vi "read_plc_datasocket.vi"() -> ()   [LabVIEW 2011]
panel:
  out "LB201_B218_ST901":string
  out "LB201_B218_ST902":string
  out "LB201_B218_SV401":string
  out "LB201_B218_GN501":string
  out "LB201_B218_GQ101":string
  out "LB201_B218_GT101":string
  out "LB201_B226_GT402":string
  out "LB201_B226_GP102":string
  out "LB201_B226_GT401":string
  out "LB201_B226_GP101":string
  out "LB201_B226_GT301":string
  out "LB201_B226_U201":string
  out "LB201_B226_GT101":string
  out "KB3_B226_U201":string
  out "KB3_B226_GT401":string
  out "KB3_B226_GP101":string
  out "KB3_B226_GT101":string
  out "VS201_B226_GT301":string
  out "VS201_B226_GP101":string
  out "VS201_B226_GT401":string
  out "VS201_B226_GT101":string
  out "VS201_B226_U201":string
  out "Elapsed Time":dbl
  out "Command":string
  out "Up Time":string
  out "Startup Time":string
  out "Version":string
  out "LB201_B230_SV201":string
  out "LB201_B230_SV401":string
  out "LB201_B230_ST902":string
  out "LB201_B230_ST901":string
  out "LB201_A213_SV201":string
  out "LB201_A213_ST902":string
  out "LB201_A235_SV401":string
  out "LB201_A235_SV201":string
  out "LB201_A235_ST902":string
  out "LB201_A235_ST901":string
  out "LB201_A225_SV401":string
  out "LB201_A225_SV201":string
  out "LB201_A225_ST902":string
  out "LB201_A225_ST901":string
  out "LB201_A213_SV401":string
  out "LB201_A213_ST901":string
  out "LB201_B230_GQ101":string
  out "LB201_B230_GT101":string
  out "LB201_A235_GQ101":string
  out "LB201_A235_GT101":string
  out "LB201_B230_GN501":string
  out "LB201_A235_GN501":string
  out "LB201_A225_GT101":string
  out "LB201_A225_GQ101":string
  out "LB201_A225_GN501":string
  out "LB201_A213_GT101":string
  out "LB201_A213_GQ101":string
  out "LB201_A213_GN501":string
  out "Deque error":errorcluster
  out "DataSocket error":errorcluster
  out "# Sent Data":u64
  # "OPC Server Status"
  # "PLC Sensing Values (Per Room)"
  # "PLC Sensing Values (Common)"
  # "PLC Actuation Values"
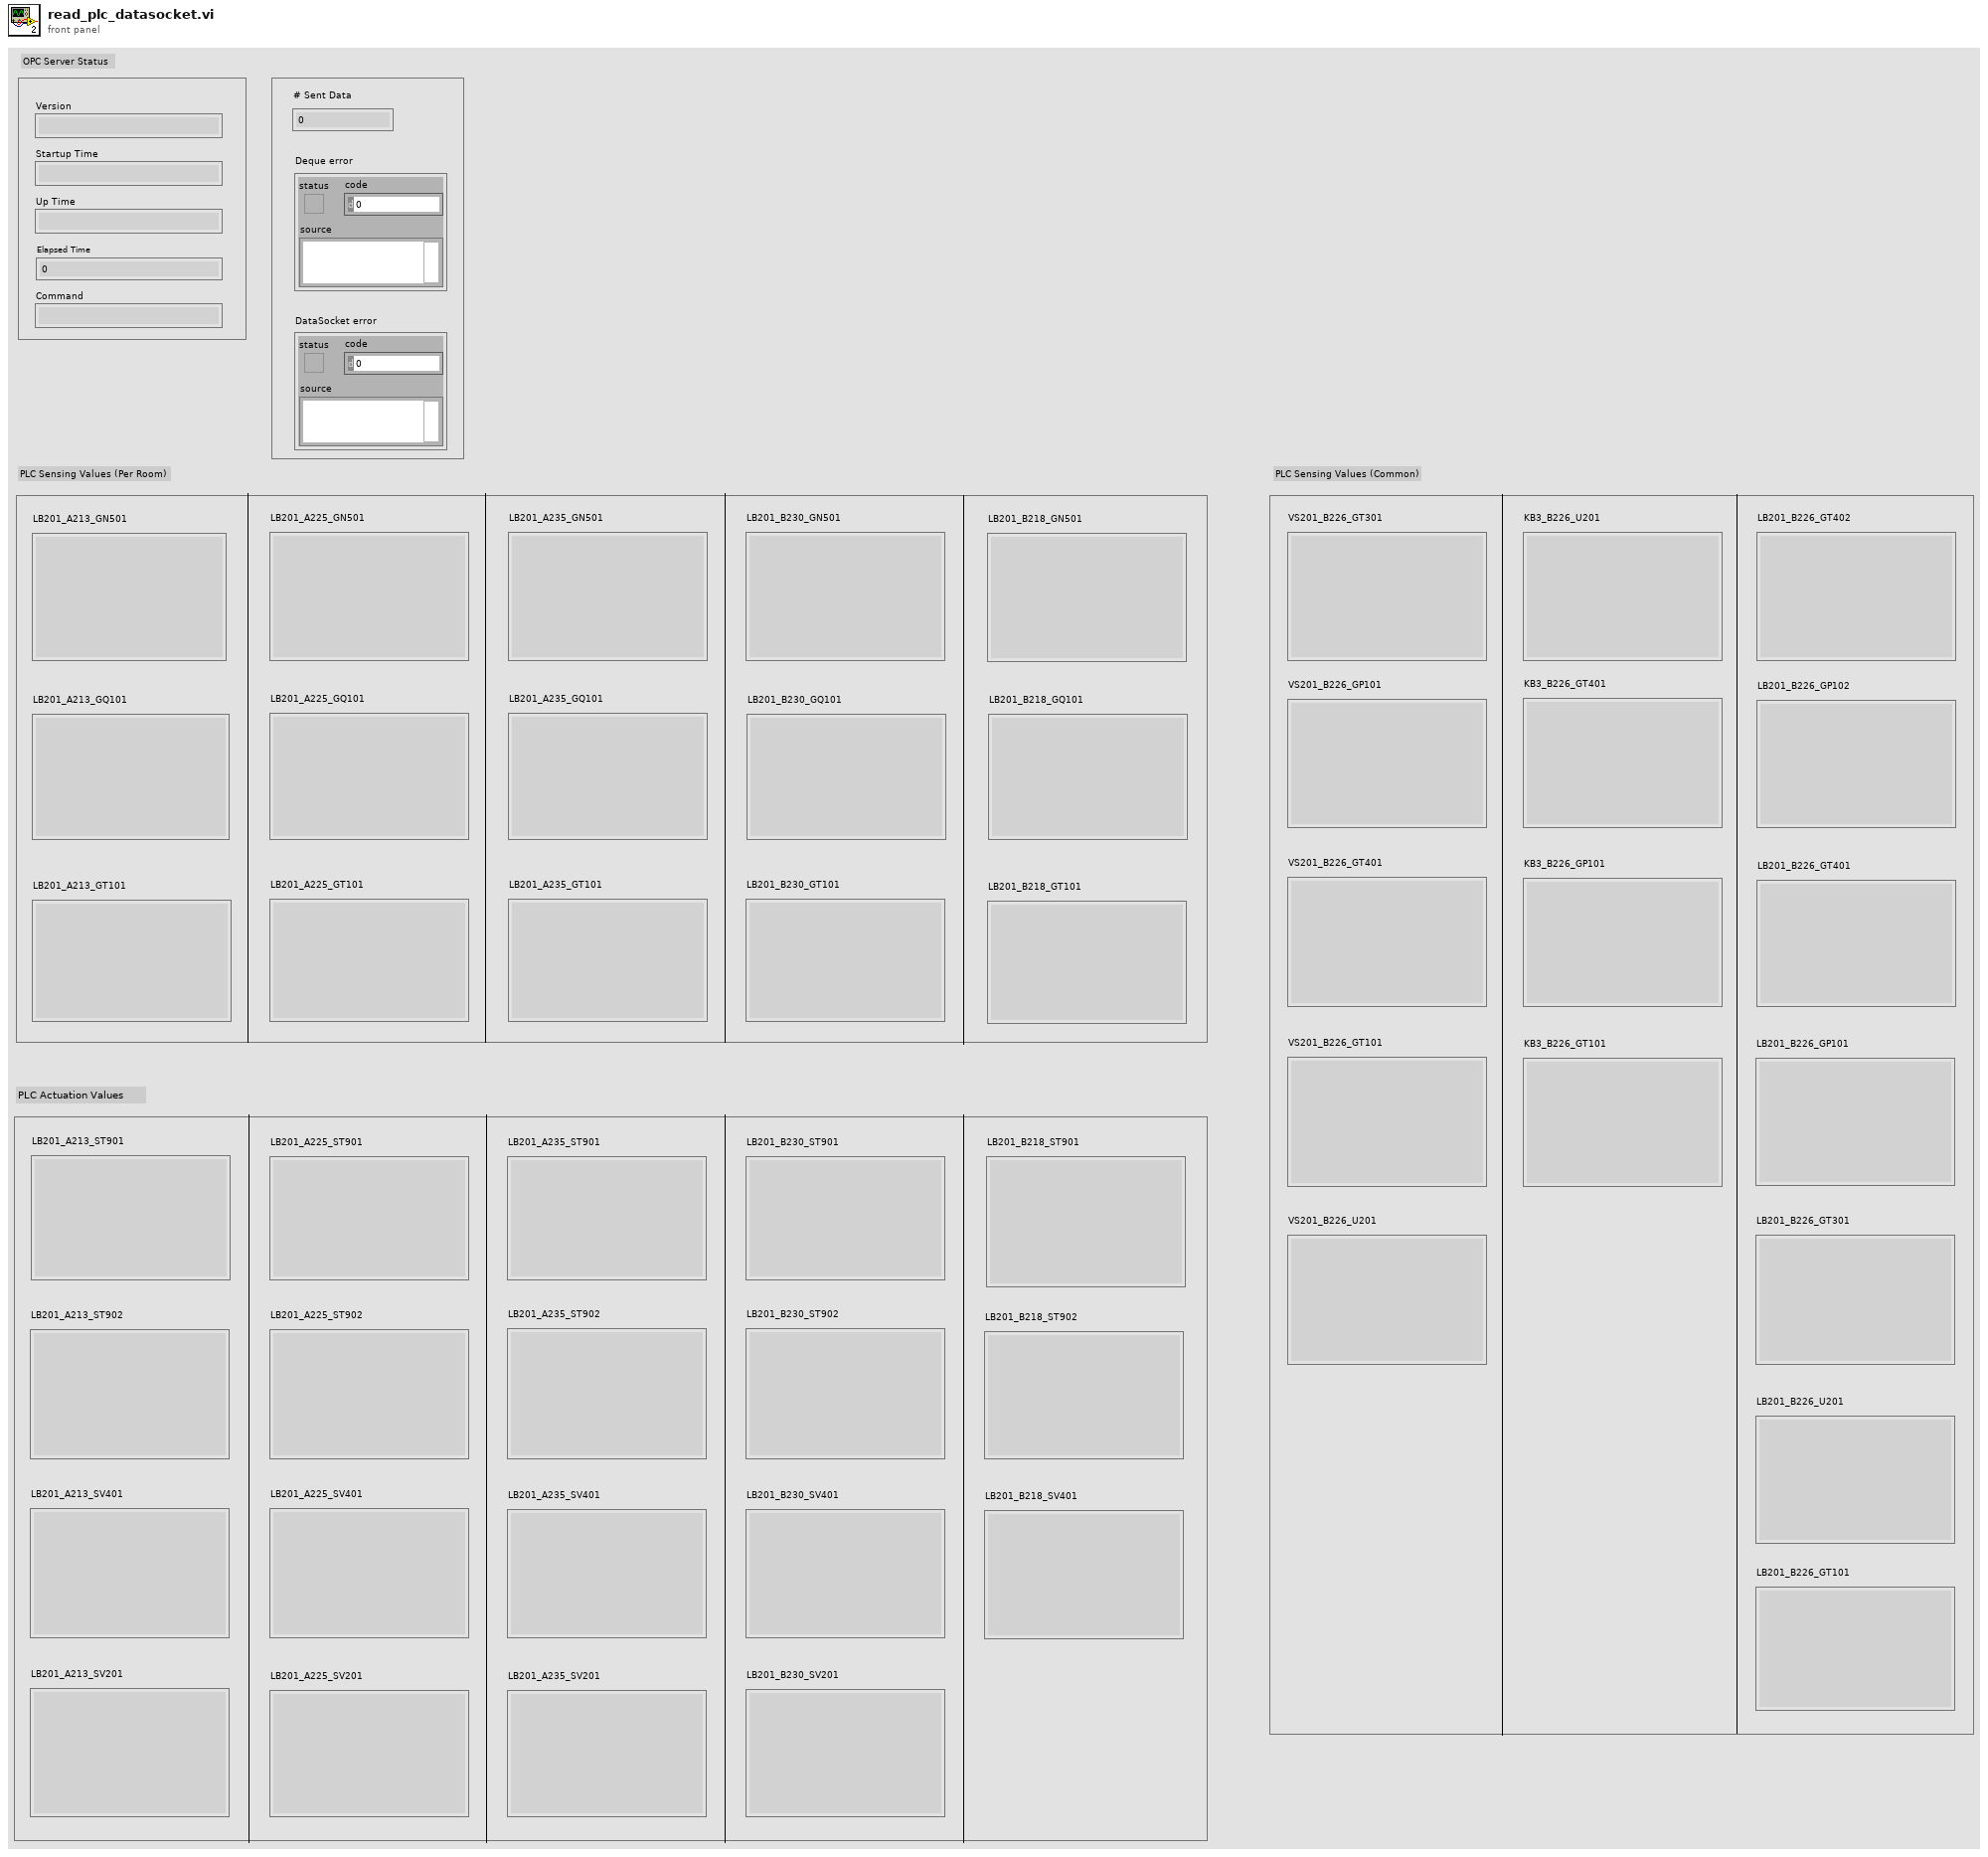
[diagram p1: front panel]
types:
  T1 = enum16{"Read", "Write", "ReadWrite", "BufferedRead", "BufferedReadWrite"}
diagram:
  w3 = string[] ["opc://localhost/Fidelix.FdxOPC/AS_KTH.AI.VS201_B226_GT301_MV.Value", "opc://localhost/Fidelix.FdxOPC/AS_KTH.AI.VS201_B226_GP101_MV.Value", "opc://localhost/Fidelix.FdxOPC/AS_KTH.AI.VS201_B226_GT401_MV.Value", "opc://localhost/Fidelix.FdxOPC/AS_KTH.AI.VS201_B226_GT101_MV.Value", "opc://localhost/Fidelix.FdxOPC/AS_KTH.AI.VS201_B226_U201_SS.Value", "opc://localhost/Fidelix.FdxOPC/AS_KTH.AI.KB3_B226_U201_SS.Value", "opc://localhost/Fidelix.FdxOPC/AS_KTH.AI.KB3_B226_GT401_MV.Value", "opc://localhost/Fidelix.FdxOPC/AS_KTH.AI.KB3_B226_GP101_MV.Value", "opc://localhost/Fidelix.FdxOPC/AS_KTH.AI.KB3_B226_GT101_MV.Value", "opc://localhost/Fidelix.FdxOPC/AS_KTH.AI.LB201_B226_GT402_MV.Value", "opc://localhost/Fidelix.FdxOPC/AS_KTH.AI.LB201_B226_GP102_MV.Value", "opc://localhost/Fidelix.FdxOPC/AS_KTH.AI.LB201_B226_GT401_MV.Value", "opc://localhost/Fidelix.FdxOPC/AS_KTH.AI.LB201_B226_GP101_MV.Value", "opc://localhost/Fidelix.FdxOPC/AS_KTH.AI.LB201_B226_GT301_MV.Value", "opc://localhost/Fidelix.FdxOPC/AS_KTH.AI.LB201_B226_U201_SS.Value", "opc://localhost/Fidelix.FdxOPC/AS_KTH.AI.LB201_B226_GT101_MV.Value"]  # Predefined items
  w32 = string[] ["opc://localhost/Fidelix.FdxOPC/AS_KTH.AI.LB201_A213_ST901_SS.Value", "opc://localhost/Fidelix.FdxOPC/AS_KTH.AI.LB201_A213_ST902_SS.Value", "opc://localhost/Fidelix.FdxOPC/AS_KTH.AI.LB201_A213_SV201_SS.Value", "opc://localhost/Fidelix.FdxOPC/AS_KTH.AI.LB201_A213_SV401_SS.Value", "opc://localhost/Fidelix.FdxOPC/AS_KTH.AI.LB201_A225_ST901_SS.Value", "opc://localhost/Fidelix.FdxOPC/AS_KTH.AI.LB201_A225_ST902_SS.Value", "opc://localhost/Fidelix.FdxOPC/AS_KTH.AI.LB201_A225_SV201_SS.Value", "opc://localhost/Fidelix.FdxOPC/AS_KTH.AI.LB201_A225_SV401_SS.Value", "opc://localhost/Fidelix.FdxOPC/AS_KTH.AI.LB201_A235_ST901_SS.Value", "opc://localhost/Fidelix.FdxOPC/AS_KTH.AI.LB201_A235_ST902_SS.Value", "opc://localhost/Fidelix.FdxOPC/AS_KTH.AI.LB201_A235_SV201_SS.Value", "opc://localhost/Fidelix.FdxOPC/AS_KTH.AI.LB201_A235_SV401_SS.Value", "opc://localhost/Fidelix.FdxOPC/AS_KTH.AI.LB201_B230_ST901_SS.Value", "opc://localhost/Fidelix.FdxOPC/AS_KTH.AI.LB201_B230_ST902_SS.Value", "opc://localhost/Fidelix.FdxOPC/AS_KTH.AI.LB201_B230_SV201_SS.Value", "opc://localhost/Fidelix.FdxOPC/AS_KTH.AI.LB201_B230_SV401_SS.Value", "opc://localhost/Fidelix.FdxOPC/AS_KTH.AI.LB201_B218_ST901_SS.Value", "opc://localhost/Fidelix.FdxOPC/AS_KTH.AI.LB201_B218_ST902_SS.Value", "opc://localhost/Fidelix.FdxOPC/AS_KTH.AI.LB201_B218_SV401_SS.Value"]  # Predefined items
  w37 = string[] ["opc://localhost/Fidelix.FdxOPC/AS_KTH.AI.LB201_A213_GN501_I.Value", "opc://localhost/Fidelix.FdxOPC/AS_KTH.AI.LB201_A213_GQ101_MV.Value", "opc://localhost/Fidelix.FdxOPC/AS_KTH.AI.LB201_A213_GT101_MV.Value", "opc://localhost/Fidelix.FdxOPC/AS_KTH.AI.LB201_A225_GN501_I.Value", "opc://localhost/Fidelix.FdxOPC/AS_KTH.AI.LB201_A225_GQ101_MV.Value", "opc://localhost/Fidelix.FdxOPC/AS_KTH.AI.LB201_A225_GT101_MV.Value", "opc://localhost/Fidelix.FdxOPC/AS_KTH.AI.LB201_A235_GN501_I.Value", "opc://localhost/Fidelix.FdxOPC/AS_KTH.AI.LB201_A235_GQ101_MV.Value", "opc://localhost/Fidelix.FdxOPC/AS_KTH.AI.LB201_A235_GT101_MV.Value", "opc://localhost/Fidelix.FdxOPC/AS_KTH.AI.LB201_B230_GN501_I.Value", "opc://localhost/Fidelix.FdxOPC/AS_KTH.AI.LB201_B230_GQ101_MV.Value", "opc://localhost/Fidelix.FdxOPC/AS_KTH.AI.LB201_B230_GT101_MV.Value", "opc://localhost/Fidelix.FdxOPC/AS_KTH.AI.LB201_B218_GN501_I.Value", "opc://localhost/Fidelix.FdxOPC/AS_KTH.AI.LB201_B218_GQ101_MV.Value", "opc://localhost/Fidelix.FdxOPC/AS_KTH.AI.LB201_B218_GT101_MV.Value"]  # Predefined items
  n1 = for {
    tunnel: w37 -> [w48] mode=indexing
    tunnel: [w47] -> w36 mode=indexing
    tunnel: [w46] -> w35 mode=indexing
    n2 = DataSocket Open(10:T1."Read" ("mode"), 11:w48) -> (0:w46:errorcluster, 3:w47:refnum<k13>)  [unwired: 1 in, 1 out]
  }
  n3 = DataSocket Open(10:T1."Read" ("mode"), 11:"opc://localhost/Fidelix.FdxOPC/ServerStatus.Version" ("URL")) -> (0:w16:errorcluster, 3:w17:refnum<k13>)  [unwired: 1 in, 1 out]
  n4 = DataSocket Open(10:T1."Read" ("mode"), 11:"opc://localhost/Fidelix.FdxOPC/ServerStatus.StartupTime" ("URL")) -> (0:w14:errorcluster, 3:w15:refnum<k13>)  [unwired: 1 in, 1 out]
  n5 = DataSocket Open(10:T1."Read" ("mode"), 11:"opc://localhost/Fidelix.FdxOPC/ServerStatus.UpTime" ("URL")) -> (0:w12:errorcluster, 3:w13:refnum<k13>)  [unwired: 1 in, 1 out]
  n6 = DataSocket Open(10:T1."Read" ("mode"), 11:"opc://localhost/Fidelix.FdxOPC/ServerStatus.ElapsedTime" ("URL")) -> (0:w10:errorcluster, 3:w11:refnum<k13>)  [unwired: 1 in, 1 out]
  n7 = DataSocket Open(10:T1."Read" ("mode"), 11:"opc://localhost/Fidelix.FdxOPC/ServerStatus.Command" ("URL")) -> (0:w8:errorcluster, 3:w9:refnum<k13>)  [unwired: 1 in, 1 out]
  n8 = while {
    tunnel: w17 -> [w58]
    tunnel: w16 -> [w57]
    tunnel: w15 -> [w56]
    tunnel: w14 -> [w55]
    tunnel: w13 -> [w54]
    tunnel: w12 -> [w53]
    tunnel: w11 -> [w52]
    tunnel: w10 -> [w51]
    tunnel: w9 -> [w50]
    tunnel: w8 -> [w49]
    stop <- TRUE continue-if-true
    n9 = DataSocket Read(8:w57, 9:100 ("ms timeout (10000)"), 10:"", 11:w58) -> (2:→"Version":string)  [unwired: 7 out]
    n10 = DataSocket Read(8:w55, 9:100 ("ms timeout (10000)"), 10:"", 11:w56) -> (2:→"Startup Time":string)  [unwired: 7 out]
    n11 = DataSocket Read(8:w53, 9:100 ("ms timeout (10000)"), 10:"", 11:w54) -> (2:→"Up Time":string)  [unwired: 7 out]
    n12 = DataSocket Read(8:w51, 9:100 ("ms timeout (10000)"), 10:0.0, 11:w52) -> (2:→"Elapsed Time":dbl)  [unwired: 7 out]
    n13 = DataSocket Read(8:w49, 9:100 ("ms timeout (10000)"), 10:"", 11:w50) -> (2:→"Command":string)  [unwired: 7 out]
    n14 = Wait Until Next ms Multiple(millisecond multiple=u32 1000) -> ()  [unwired: 1 out]
  }
  n15 = Obtain Queue(max queue size (-1, unlimited)=-1, name (unnamed)="SendingQuePLC", element data type="") -> (queue out=w2:refnum<queue>, error out=w1:errorcluster)  [unwired: 2 in, 1 out]
  n16 = while {
    tunnel: w1 -> [w322]
    tunnel: w2 -> [w321]
    tunnel: w36 -> [w250]
    tunnel: w35 -> [w249]
    tunnel: [w247] -> w34
    tunnel: [w246] -> w33
    stop <- TRUE continue-if-true
    w117 = "\r"
    w116 = "\r"
    w115 = "\r"
    w142 = "\r"
    w154 = "\r"
    w166 = "\r"
    w178 = "\r"
    w190 = "\r"
    w125 = "\r"
    w126 = "\r"
    w127 = "\r"
    w128 = "\r"
    w129 = "\r"
    w130 = "\r"
    w191 = "\r"
    # "PLC Sensing Values (Per Room)"
    n17 = for {
      tunnel: w250 -> [w328] mode=indexing
      tunnel: [w330] -> w247 mode=indexing
      tunnel: w249 -> [w327] mode=indexing
      tunnel: [w325] -> w248 mode=indexing
      tunnel: [w329] -> w246 mode=indexing
      n18 = DataSocket Read(8:w327, 9:500 ("ms timeout (10000)"), 10:0.0, 11:w328) -> (0:w329:errorcluster, 2:w325:dbl, 3:w330:refnum<k13>)  [unwired: 5 out]
    }
    n19 = Build Array(w248) -> (w118:dbl[][])
    n20 = Index Array(array=w118, index (row)=0, index (col)=12 ("disabled index (col)")) -> (element=w78:dbl)
    n21 = Index Array(array=w118, index (row)=0, index (col)=13 ("disabled index (col)")) -> (element=w77:dbl)
    n22 = Index Array(array=w118, index (row)=0, index (col)=14 ("disabled index (col)")) -> (element=w76:dbl)
    n23 = Index Array(array=w118, index (row)=0, index (col)=0 ("disabled index (col)")) -> (element=w237:dbl)
    n24 = Index Array(array=w118, index (row)=0, index (col)=1 ("disabled index (col)")) -> (element=w179:dbl)
    n25 = Index Array(array=w118, index (row)=0, index (col)=2 ("disabled index (col)")) -> (element=w167:dbl)
    n26 = Index Array(array=w118, index (row)=0, index (col)=3 ("disabled index (col)")) -> (element=w155:dbl)
    n27 = Index Array(array=w118, index (row)=0, index (col)=4 ("disabled index (col)")) -> (element=w143:dbl)
    n28 = Index Array(array=w118, index (row)=0, index (col)=5 ("disabled index (col)")) -> (element=w131:dbl)
    n29 = Index Array(array=w118, index (row)=0, index (col)=6 ("disabled index (col)")) -> (element=w220:dbl)
    n30 = Index Array(array=w118, index (row)=0, index (col)=7 ("disabled index (col)")) -> (element=w219:dbl)
    n31 = Index Array(array=w118, index (row)=0, index (col)=8 ("disabled index (col)")) -> (element=w218:dbl)
    n32 = Index Array(array=w118, index (row)=0, index (col)=9 ("disabled index (col)")) -> (element=w217:dbl)
    n33 = Index Array(array=w118, index (row)=0, index (col)=10 ("disabled index (col)")) -> (element=w216:dbl)
    n34 = Index Array(array=w118, index (row)=0, index (col)=11 ("disabled index (col)")) -> (element=w215:dbl)
    n35 = Wait Until Next ms Multiple(millisecond multiple=u32 30000) -> ()  [unwired: 1 out]
    n36 = Number To Fractional String(number=w143, precision (6)=i16 2) -> (F-format string=w146:string)  [unwired: 2 in]
    n37 = Number To Fractional String(number=w167, precision (6)=i16 2) -> (F-format string=w170:string)  [unwired: 2 in]
    n38 = Format Date/Time String(time format string (%c)="%y%m%d%H%M%S") -> (date/time string=w171:string)  [unwired: 2 in]
    n39 = Number To Fractional String(number=w179, precision (6)=i16 2) -> (F-format string=w182:string)  [unwired: 2 in]
    n40 = Format Date/Time String(time format string (%c)="%y%m%d%H%M%S") -> (date/time string=w183:string)  [unwired: 2 in]
    n41 = Number To Fractional String(number=w131, precision (6)=i16 2) -> (F-format string=w134:string)  [unwired: 2 in]
    n42 = Number To Fractional String(number=w155, precision (6)=i16 2) -> (F-format string=w158:string)  [unwired: 2 in]
    n43 = Format Date/Time String(time format string (%c)="%y%m%d%H%M%S") -> (date/time string=w159:string)  [unwired: 2 in]
    n44 = Number To Fractional String(number=w237, precision (6)=i16 2) -> (F-format string=w317:string)  [unwired: 2 in]
    n45 = Format Date/Time String(time format string (%c)="%y%m%d%H%M%S") -> (date/time string=w316:string)  [unwired: 2 in]
    n46 = Number To Fractional String(number=w220, precision (6)=i16 2) -> (F-format string=w308:string)  [unwired: 2 in]
    n47 = Number To Fractional String(number=w218, precision (6)=i16 2) -> (F-format string=w294:string)  [unwired: 2 in]
    n48 = Number To Fractional String(number=w219, precision (6)=i16 2) -> (F-format string=w285:string)  [unwired: 2 in]
    n49 = Number To Fractional String(number=w217, precision (6)=i16 2) -> (F-format string=w299:string)  [unwired: 2 in]
    n50 = Number To Fractional String(number=w78, precision (6)=i16 2) -> (F-format string=w85:string)  [unwired: 2 in]
    n51 = Number To Fractional String(number=w215, precision (6)=i16 2) -> (F-format string=w271:string)  [unwired: 2 in]
    n52 = Number To Fractional String(number=w216, precision (6)=i16 2) -> (F-format string=w280:string)  [unwired: 2 in]
    n53 = Number To Fractional String(number=w76, precision (6)=i16 2) -> (F-format string=w99:string)  [unwired: 2 in]
    n54 = Number To Fractional String(number=w77, precision (6)=i16 2) -> (F-format string=w90:string)  [unwired: 2 in]
    n55 = Format Date/Time String(time format string (%c)="%y%m%d%H%M%S") -> (date/time string=w147:string)  [unwired: 2 in]
    n56 = Format Date/Time String(time format string (%c)="%y%m%d%H%M%S") -> (date/time string=w295:string)  [unwired: 2 in]
    n57 = Format Date/Time String(time format string (%c)="%y%m%d%H%M%S") -> (date/time string=w284:string)  [unwired: 2 in]
    n58 = Format Date/Time String(time format string (%c)="%y%m%d%H%M%S") -> (date/time string=w135:string)  [unwired: 2 in]
    n59 = Format Date/Time String(time format string (%c)="%y%m%d%H%M%S") -> (date/time string=w298:string)  [unwired: 2 in]
    n60 = Format Date/Time String(time format string (%c)="%y%m%d%H%M%S") -> (date/time string=w86:string)  [unwired: 2 in]
    n61 = Format Date/Time String(time format string (%c)="%y%m%d%H%M%S") -> (date/time string=w270:string)  [unwired: 2 in]
    n62 = Format Date/Time String(time format string (%c)="%y%m%d%H%M%S") -> (date/time string=w281:string)  [unwired: 2 in]
    n63 = Format Date/Time String(time format string (%c)="%y%m%d%H%M%S") -> (date/time string=w100:string)  [unwired: 2 in]
    n64 = Format Date/Time String(time format string (%c)="%y%m%d%H%M%S") -> (date/time string=w89:string)  [unwired: 2 in]
    n65 = Format Date/Time String(time format string (%c)="%y%m%d%H%M%S") -> (date/time string=w309:string)  [unwired: 2 in]
    n66 = Concatenate Strings("2002" ("string"), w154, "C" ("string"), w154, "30" ("string"), w154, w146, w154, w147, w154, "LB201_A225", w154, "0.3145 0.3240 0.5" ("string")) -> (w144:string)
    "LB201_A225_GQ101" <- w144
    n67 = Concatenate Strings("2001" ("string"), w178, "T" ("string"), w178, "10" ("string"), w178, w170, w178, w171, w178, "LB201_A213", w178, "0.5524 0.3240 0.5" ("string")) -> (w168:string)
    "LB201_A213_GT101" <- w168
    n68 = Concatenate Strings("2001" ("string"), w190, "C" ("string"), w190, "30" ("string"), w190, w182, w190, w183, w190, "LB201_A213", w190, "0.5524 0.3240 0.5" ("string")) -> (w180:string)
    "LB201_A213_GQ101" <- w180
    n69 = Concatenate Strings("2002" ("string"), w142, "T" ("string"), w142, "10" ("string"), w142, w134, w142, w135, w142, "LB201_A225", w142, "0.3145 0.3240 0.5" ("string")) -> (w132:string)
    "LB201_A225_GT101" <- w132
    n70 = Concatenate Strings("2002" ("string"), w166, "M" ("string"), w166, "51" ("string"), w166, w158, w166, w159, w166, "LB201_A225", w166, "0.3145 0.3240 0.5" ("string")) -> (w156:string)
    "LB201_A225_GN501" <- w156
    n71 = Concatenate Strings("2001" ("string"), w191, "M" ("string"), w191, "51" ("string"), w191, w317, w191, w316, w191, "LB201_A213", w191, "0.5524 0.3240 0.5" ("string")) -> (w320:string)
    "LB201_A213_GN501" <- w320
    n72 = Concatenate Strings("2003" ("string"), w130, "M" ("string"), w130, "51" ("string"), w130, w308, w130, w309, w130, "LB201_A235", w130, "0.1735 0.3240 0.5" ("string")) -> (w305:string)
    "LB201_A235_GN501" <- w305
    n73 = Concatenate Strings("2003" ("string"), w128, "T" ("string"), w128, "10" ("string"), w128, w294, w128, w295, w128, "LB201_A235", w128, "0.1735 0.3240 0.5" ("string")) -> (w291:string)
    "LB201_A235_GT101" <- w291
    n74 = Concatenate Strings("2003" ("string"), w129, "C" ("string"), w129, "30" ("string"), w129, w285, w129, w284, w129, "LB201_A235", w129, "0.1735 0.3240 0.5" ("string")) -> (w288:string)
    "LB201_A235_GQ101" <- w288
    n75 = Concatenate Strings("2004" ("string"), w127, "M" ("string"), w127, "51" ("string"), w127, w299, w127, w298, w127, "LB201_B230", w127, "0.2761 0.6773 0.5" ("string")) -> (w302:string)
    "LB201_B230_GN501" <- w302
    n76 = Concatenate Strings("2005" ("string"), w115, "M" ("string"), w115, "51" ("string"), w115, w85, w115, w86, w115, "LB201_B218", w115, "0.5844 0.6607 0.5" ("string")) -> (w82:string)
    "LB201_B218_GN501" <- w82
    n77 = Concatenate Strings("2004" ("string"), w125, "T" ("string"), w125, "10" ("string"), w125, w271, w125, w270, w125, "LB201_B230", w125, "0.2761 0.6773 0.5" ("string")) -> (w274:string)
    "LB201_B230_GT101" <- w274
    n78 = Concatenate Strings("2004" ("string"), w126, "C" ("string"), w126, "30" ("string"), w126, w280, w126, w281, w126, "LB201_B230", w126, "0.2761 0.6773 0.5" ("string")) -> (w277:string)
    "LB201_B230_GQ101" <- w277
    n79 = Concatenate Strings("2005" ("string"), w117, "T" ("string"), w117, "10" ("string"), w117, w99, w117, w100, w117, "LB201_B218", w117, "0.5844 0.6607 0.5" ("string")) -> (w96:string)
    "LB201_B218_GT101" <- w96
    n80 = Concatenate Strings("2005" ("string"), w116, "C" ("string"), w116, "30" ("string"), w116, w90, w116, w89, w116, "LB201_B218", w116, "0.5844 0.6607 0.5" ("string")) -> (w93:string)
    "LB201_B218_GQ101" <- w93
    n81 = Enqueue Element(queue=w321, element=w320, error in (no error)=w322) -> (queue out=w314:refnum<queue>, error out=w312:errorcluster)  [unwired: 1 in, 1 out]
    n82 = Enqueue Element(queue=w314, element=w180, error in (no error)=w312) -> (queue out=w313:refnum<queue>, error out=w311:errorcluster)  [unwired: 1 in, 1 out]
    n83 = Enqueue Element(queue=w313, element=w168, error in (no error)=w311) -> (queue out=w268:refnum<queue>, error out=w267:errorcluster)  [unwired: 1 in, 1 out]
    n84 = Enqueue Element(queue=w268, element=w156, error in (no error)=w267) -> (queue out=w266:refnum<queue>, error out=w265:errorcluster)  [unwired: 1 in, 1 out]
    n85 = Enqueue Element(queue=w266, element=w144, error in (no error)=w265) -> (queue out=w264:refnum<queue>, error out=w263:errorcluster)  [unwired: 1 in, 1 out]
    n86 = Enqueue Element(queue=w264, element=w132, error in (no error)=w263) -> (queue out=w262:refnum<queue>, error out=w261:errorcluster)  [unwired: 1 in, 1 out]
    n87 = Enqueue Element(queue=w262, element=w305, error in (no error)=w261) -> (queue out=w260:refnum<queue>, error out=w259:errorcluster)  [unwired: 1 in, 1 out]
    n88 = Enqueue Element(queue=w260, element=w288, error in (no error)=w259) -> (queue out=w258:refnum<queue>, error out=w257:errorcluster)  [unwired: 1 in, 1 out]
    n89 = Enqueue Element(queue=w258, element=w291, error in (no error)=w257) -> (queue out=w256:refnum<queue>, error out=w255:errorcluster)  [unwired: 1 in, 1 out]
    n90 = Enqueue Element(queue=w256, element=w302, error in (no error)=w255) -> (queue out=w254:refnum<queue>, error out=w253:errorcluster)  [unwired: 1 in, 1 out]
    n91 = Enqueue Element(queue=w254, element=w277, error in (no error)=w253) -> (queue out=w252:refnum<queue>, error out=w251:errorcluster)  [unwired: 1 in, 1 out]
    n92 = Enqueue Element(queue=w252, element=w274, error in (no error)=w251) -> (queue out=w80:refnum<queue>, error out=w79:errorcluster)  [unwired: 1 in, 1 out]
    n93 = Enqueue Element(queue=w80, element=w82, error in (no error)=w79) -> (queue out=w102:refnum<queue>, error out=w103:errorcluster)  [unwired: 1 in, 1 out]
    n94 = Enqueue Element(queue=w102, element=w93, error in (no error)=w103) -> (queue out=w104:refnum<queue>, error out=w105:errorcluster)  [unwired: 1 in, 1 out]
    n95 = Enqueue Element(queue=w104, element=w96, error in (no error)=w105) -> ()  [unwired: 1 in, 3 out]
  }
  n96 = for {
    tunnel: w34 -> [w332] mode=indexing
    tunnel: w33 -> [w331] mode=indexing
    n97 = DataSocket Close(8:w331, 11:w332) -> ()  [unwired: 3 out]
  }
  n98 = DataSocket Open(10:T1."Write" ("mode"), 11:"dstp://localhost/plcs" ("URL 3")) -> (0:w39:errorcluster, 3:w40:refnum<k13>)  [unwired: 2 in]
  n99 = while {
    tunnel: w2 -> [w345]
    tunnel: w40 -> [w344]
    tunnel: w39 -> [w339]
    i -> [w337]
    stop <- w338 stop-if-true
    n100 = Dequeue Element(queue=w345) -> (element=w342:string, error out=w341:errorcluster)  [unwired: 2 in, 2 out]
    "Deque error" <- w341
    n101 = To Variant(anything=w342) -> (Variant=w343:variant)
    n102 = DataSocket Write(8:w339, 10:w343, 11:w344) -> (0:w340:errorcluster)  [unwired: 3 out]
    "DataSocket error" <- w340
    n103 = Unbundle By Name(w340) -> ("status"=w334:bool)
    n104 = Unbundle By Name(w341) -> ("status"=w333:bool)
    n105 = Compound Arithmetic op=OR(w334, w333) -> (w338:bool)
    n106 = call "logging.vi"("data"="counter.vi: datasocket error.", "Boolean"=w334) -> ()  [unwired: 1 in]
    n107 = call "logging.vi"("data"="counter.vi: deque error.", "Boolean"=w333) -> ()  [unwired: 1 in]
    "# Sent Data" <- w337
  }
  n108 = for {
    tunnel: w3 -> [w349] mode=indexing
    tunnel: [w348] -> w4 mode=indexing
    tunnel: [w347] -> w5 mode=indexing
    n109 = DataSocket Open(10:T1."Read" ("mode"), 11:w349) -> (0:w347:errorcluster, 3:w348:refnum<k13>)  [unwired: 1 in, 1 out]
  }
  n110 = while {
    tunnel: w4 -> [w611]
    tunnel: w5 -> [w610]
    tunnel: [w608] -> w6
    tunnel: [w607] -> w7
    tunnel: w2 -> [w565]
    tunnel: w1 -> [w564]
    stop <- TRUE continue-if-true
    w361 = "\r"
    w374 = "\r"
    w385 = "\r"
    w397 = "\r"
    w409 = "\r"
    w421 = "\r"
    w433 = "\r"
    w445 = "\r"
    w457 = "\r"
    w469 = "\r"
    w481 = "\r"
    w493 = "\r"
    w505 = "\r"
    w518 = "\r"
    w529 = "\r"
    w541 = "\r"
    # "PLC Sensing Values (Common)"
    n111 = for {
      tunnel: w611 -> [w618] mode=indexing
      tunnel: [w620] -> w608 mode=indexing
      tunnel: w610 -> [w617] mode=indexing
      tunnel: [w615] -> w609 mode=indexing
      tunnel: [w619] -> w607 mode=indexing
      n112 = DataSocket Read(8:w617, 9:500 ("ms timeout (10000)"), 10:0.0, 11:w618) -> (0:w619:errorcluster, 2:w615:dbl, 3:w620:refnum<k13>)  [unwired: 5 out]
    }
    n113 = Build Array(w609) -> (w574:dbl[][])
    n114 = Index Array(array=w574, index (row)=0, index (col)=0 ("disabled index (col)")) -> (element=w530:dbl)
    n115 = Index Array(array=w574, index (row)=0, index (col)=1 ("disabled index (col)")) -> (element=w507:dbl)
    n116 = Index Array(array=w574, index (row)=0, index (col)=2 ("disabled index (col)")) -> (element=w506:dbl)
    n117 = Index Array(array=w574, index (row)=0, index (col)=3 ("disabled index (col)")) -> (element=w494:dbl)
    n118 = Index Array(array=w574, index (row)=0, index (col)=4 ("disabled index (col)")) -> (element=w482:dbl)
    n119 = Index Array(array=w574, index (row)=0, index (col)=5 ("disabled index (col)")) -> (element=w470:dbl)
    n120 = Index Array(array=w574, index (row)=0, index (col)=6 ("disabled index (col)")) -> (element=w458:dbl)
    n121 = Index Array(array=w574, index (row)=0, index (col)=7 ("disabled index (col)")) -> (element=w446:dbl)
    n122 = Index Array(array=w574, index (row)=0, index (col)=8 ("disabled index (col)")) -> (element=w434:dbl)
    n123 = Index Array(array=w574, index (row)=0, index (col)=9 ("disabled index (col)")) -> (element=w422:dbl)
    n124 = Index Array(array=w574, index (row)=0, index (col)=10 ("disabled index (col)")) -> (element=w410:dbl)
    n125 = Index Array(array=w574, index (row)=0, index (col)=11 ("disabled index (col)")) -> (element=w398:dbl)
    n126 = Index Array(array=w574, index (row)=0, index (col)=12 ("disabled index (col)")) -> (element=w386:dbl)
    n127 = Index Array(array=w574, index (row)=0, index (col)=13 ("disabled index (col)")) -> (element=w362:dbl)
    n128 = Index Array(array=w574, index (row)=0, index (col)=14 ("disabled index (col)")) -> (element=w363:dbl)
    n129 = Index Array(array=w574, index (row)=0, index (col)=15 ("disabled index (col)")) -> (element=w350:dbl)
    n130 = Wait Until Next ms Multiple(millisecond multiple=u32 30000) -> ()  [unwired: 1 out]
    n131 = Number To Fractional String(number=w507, precision (6)=i16 2) -> (F-format string=w522:string)  [unwired: 2 in]
    n132 = Number To Fractional String(number=w530, precision (6)=i16 2) -> (F-format string=w534:string)  [unwired: 2 in]
    n133 = Number To Fractional String(number=w494, precision (6)=i16 2) -> (F-format string=w498:string)  [unwired: 2 in]
    n134 = Number To Fractional String(number=w506, precision (6)=i16 2) -> (F-format string=w511:string)  [unwired: 2 in]
    n135 = Number To Fractional String(number=w482, precision (6)=i16 2) -> (F-format string=w486:string)  [unwired: 2 in]
    n136 = Number To Fractional String(number=w458, precision (6)=i16 2) -> (F-format string=w462:string)  [unwired: 2 in]
    n137 = Number To Fractional String(number=w470, precision (6)=i16 2) -> (F-format string=w474:string)  [unwired: 2 in]
    n138 = Number To Fractional String(number=w434, precision (6)=i16 2) -> (F-format string=w438:string)  [unwired: 2 in]
    n139 = Number To Fractional String(number=w446, precision (6)=i16 2) -> (F-format string=w450:string)  [unwired: 2 in]
    n140 = Number To Fractional String(number=w410, precision (6)=i16 2) -> (F-format string=w414:string)  [unwired: 2 in]
    n141 = Number To Fractional String(number=w422, precision (6)=i16 2) -> (F-format string=w426:string)  [unwired: 2 in]
    n142 = Number To Fractional String(number=w398, precision (6)=i16 2) -> (F-format string=w402:string)  [unwired: 2 in]
    n143 = Number To Fractional String(number=w386, precision (6)=i16 2) -> (F-format string=w390:string)  [unwired: 2 in]
    n144 = Number To Fractional String(number=w350, precision (6)=i16 2) -> (F-format string=w355:string)  [unwired: 2 in]
    n145 = Number To Fractional String(number=w362, precision (6)=i16 2) -> (F-format string=w379:string)  [unwired: 2 in]
    n146 = Number To Fractional String(number=w363, precision (6)=i16 2) -> (F-format string=w368:string)  [unwired: 2 in]
    n147 = Format Date/Time String(time format string (%c)="%y%m%d%H%M%S") -> (date/time string=w521:string)  [unwired: 2 in]
    n148 = Format Date/Time String(time format string (%c)="%y%m%d%H%M%S") -> (date/time string=w533:string)  [unwired: 2 in]
    n149 = Format Date/Time String(time format string (%c)="%y%m%d%H%M%S") -> (date/time string=w497:string)  [unwired: 2 in]
    n150 = Format Date/Time String(time format string (%c)="%y%m%d%H%M%S") -> (date/time string=w510:string)  [unwired: 2 in]
    n151 = Format Date/Time String(time format string (%c)="%y%m%d%H%M%S") -> (date/time string=w485:string)  [unwired: 2 in]
    n152 = Format Date/Time String(time format string (%c)="%y%m%d%H%M%S") -> (date/time string=w461:string)  [unwired: 2 in]
    n153 = Format Date/Time String(time format string (%c)="%y%m%d%H%M%S") -> (date/time string=w473:string)  [unwired: 2 in]
    n154 = Format Date/Time String(time format string (%c)="%y%m%d%H%M%S") -> (date/time string=w437:string)  [unwired: 2 in]
    n155 = Format Date/Time String(time format string (%c)="%y%m%d%H%M%S") -> (date/time string=w449:string)  [unwired: 2 in]
    n156 = Format Date/Time String(time format string (%c)="%y%m%d%H%M%S") -> (date/time string=w413:string)  [unwired: 2 in]
    n157 = Format Date/Time String(time format string (%c)="%y%m%d%H%M%S") -> (date/time string=w425:string)  [unwired: 2 in]
    n158 = Format Date/Time String(time format string (%c)="%y%m%d%H%M%S") -> (date/time string=w401:string)  [unwired: 2 in]
    n159 = Format Date/Time String(time format string (%c)="%y%m%d%H%M%S") -> (date/time string=w389:string)  [unwired: 2 in]
    n160 = Format Date/Time String(time format string (%c)="%y%m%d%H%M%S") -> (date/time string=w354:string)  [unwired: 2 in]
    n161 = Format Date/Time String(time format string (%c)="%y%m%d%H%M%S") -> (date/time string=w378:string)  [unwired: 2 in]
    n162 = Format Date/Time String(time format string (%c)="%y%m%d%H%M%S") -> (date/time string=w367:string)  [unwired: 2 in]
    n163 = Concatenate Strings("2000" ("string"), w529, "P" ("string"), w529, "507" ("string"), w529, w522, w529, w521, w529, "VS201_B226", w529, "0.4619 0.6696 0.5" ("string")) -> (w519:string)
    "VS201_B226_GP101" <- w519
    n164 = Concatenate Strings("2000" ("string"), w541, "T" ("string"), w541, "19" ("string"), w541, w534, w541, w533, w541, "VS201_B226", w541, "0.4619 0.6696 0.5" ("string")) -> (w531:string)
    "VS201_B226_GT301" <- w531
    n165 = Concatenate Strings("2000" ("string"), w505, "T" ("string"), w505, "521" ("string"), w505, w498, w505, w497, w505, "VS201_B226", w505, "0.4619 0.6696 0.5" ("string")) -> (w495:string)
    "VS201_B226_GT101" <- w495
    n166 = Concatenate Strings("2000" ("string"), w518, "T" ("string"), w518, "522" ("string"), w518, w511, w518, w510, w518, "VS201_B226", w518, "0.4619 0.6696 0.5" ("string")) -> (w508:string)
    "VS201_B226_GT401" <- w508
    n167 = Concatenate Strings("2000" ("string"), w493, "V" ("string"), w493, "512" ("string"), w493, w486, w493, w485, w493, "VS201_B226", w493, "0.4619 0.6696 0.5" ("string")) -> (w483:string)
    "VS201_B226_U201" <- w483
    n168 = Concatenate Strings("2000" ("string"), w469, "T" ("string"), w469, "524" ("string"), w469, w462, w469, w461, w469, "KB3_B226", w469, "0.4619 0.6696 0.5" ("string")) -> (w459:string)
    "KB3_B226_GT401" <- w459
    n169 = Concatenate Strings("2000" ("string"), w481, "V" ("string"), w481, "513" ("string"), w481, w474, w481, w473, w481, "KB3_B226", w481, "0.4619 0.6696 0.5" ("string")) -> (w471:string)
    "KB3_B226_U201" <- w471
    n170 = Concatenate Strings("2000" ("string"), w445, "T" ("string"), w445, "523" ("string"), w445, w438, w445, w437, w445, "KB3_B226", w445, "0.4619 0.6696 0.5" ("string")) -> (w435:string)
    "KB3_B226_GT101" <- w435
    n171 = Concatenate Strings("2000" ("string"), w457, "P" ("string"), w457, "508" ("string"), w457, w450, w457, w449, w457, "KB3_B226", w457, "0.4619 0.6696 0.5" ("string")) -> (w447:string)
    "KB3_B226_GP101" <- w447
    n172 = Concatenate Strings("2000" ("string"), w421, "P" ("string"), w421, "506" ("string"), w421, w414, w421, w413, w421, "LB201_B226", w421, "0.4619 0.6696 0.5" ("string")) -> (w411:string)
    "LB201_B226_GP102" <- w411
    n173 = Concatenate Strings("2000" ("string"), w433, "T" ("string"), w433, "504" ("string"), w433, w426, w433, w425, w433, "LB201_B226", w433, "0.4619 0.6696 0.5" ("string")) -> (w423:string)
    "LB201_B226_GT402" <- w423
    n174 = Concatenate Strings("2000" ("string"), w409, "T" ("string"), w409, "503" ("string"), w409, w402, w409, w401, w409, "LB201_B226", w409, "0.4619 0.6696 0.5" ("string")) -> (w399:string)
    "LB201_B226_GT401" <- w399
    n175 = Concatenate Strings("2000" ("string"), w397, "P" ("string"), w397, "505" ("string"), w397, w390, w397, w389, w397, "LB201_B226", w397, "0.4619 0.6696 0.5" ("string")) -> (w387:string)
    "LB201_B226_GP101" <- w387
    n176 = Concatenate Strings("2000" ("string"), w361, "T" ("string"), w361, "501" ("string"), w361, w355, w361, w354, w361, "LB201_B226", w361, "0.4619 0.6696 0.5" ("string")) -> (w351:string)
    "LB201_B226_GT101" <- w351
    n177 = Concatenate Strings("2000" ("string"), w385, "T" ("string"), w385, "502" ("string"), w385, w379, w385, w378, w385, "LB201_B226", w385, "0.4619 0.6696 0.5" ("string")) -> (w376:string)
    "LB201_B226_GT301" <- w376
    n178 = Concatenate Strings("2000" ("string"), w374, "V" ("string"), w374, "511" ("string"), w374, w368, w374, w367, w374, "LB201_B226", w374, "0.4619 0.6696 0.5" ("string")) -> (w364:string)
    "LB201_B226_U201" <- w364
    n179 = Enqueue Element(queue=w565, element=w531, error in (no error)=w564) -> (queue out=w566:refnum<queue>, error out=w567:errorcluster)  [unwired: 1 in, 1 out]
    n180 = Enqueue Element(queue=w566, element=w519, error in (no error)=w567) -> (queue out=w568:refnum<queue>, error out=w569:errorcluster)  [unwired: 1 in, 1 out]
    n181 = Enqueue Element(queue=w568, element=w508, error in (no error)=w569) -> (queue out=w570:refnum<queue>, error out=w571:errorcluster)  [unwired: 1 in, 1 out]
    n182 = Enqueue Element(queue=w570, element=w495, error in (no error)=w571) -> (queue out=w572:refnum<queue>, error out=w573:errorcluster)  [unwired: 1 in, 1 out]
    n183 = Enqueue Element(queue=w572, element=w483, error in (no error)=w573) -> (queue out=w557:refnum<queue>, error out=w556:errorcluster)  [unwired: 1 in, 1 out]
    n184 = Enqueue Element(queue=w557, element=w471, error in (no error)=w556) -> (queue out=w563:refnum<queue>, error out=w562:errorcluster)  [unwired: 1 in, 1 out]
    n185 = Enqueue Element(queue=w563, element=w459, error in (no error)=w562) -> (queue out=w561:refnum<queue>, error out=w560:errorcluster)  [unwired: 1 in, 1 out]
    n186 = Enqueue Element(queue=w561, element=w447, error in (no error)=w560) -> (queue out=w559:refnum<queue>, error out=w558:errorcluster)  [unwired: 1 in, 1 out]
    n187 = Enqueue Element(queue=w559, element=w435, error in (no error)=w558) -> (queue out=w542:refnum<queue>, error out=w543:errorcluster)  [unwired: 1 in, 1 out]
    n188 = Enqueue Element(queue=w542, element=w423, error in (no error)=w543) -> (queue out=w547:refnum<queue>, error out=w546:errorcluster)  [unwired: 1 in, 1 out]
    n189 = Enqueue Element(queue=w547, element=w411, error in (no error)=w546) -> (queue out=w545:refnum<queue>, error out=w544:errorcluster)  [unwired: 1 in, 1 out]
    n190 = Enqueue Element(queue=w545, element=w399, error in (no error)=w544) -> (queue out=w554:refnum<queue>, error out=w555:errorcluster)  [unwired: 1 in, 1 out]
    n191 = Enqueue Element(queue=w554, element=w387, error in (no error)=w555) -> (queue out=w548:refnum<queue>, error out=w549:errorcluster)  [unwired: 1 in, 1 out]
    n192 = Enqueue Element(queue=w548, element=w376, error in (no error)=w549) -> (queue out=w550:refnum<queue>, error out=w551:errorcluster)  [unwired: 1 in, 1 out]
    n193 = Enqueue Element(queue=w550, element=w364, error in (no error)=w551) -> (queue out=w552:refnum<queue>, error out=w553:errorcluster)  [unwired: 1 in, 1 out]
    n194 = Enqueue Element(queue=w552, element=w351, error in (no error)=w553) -> ()  [unwired: 1 in, 3 out]
  }
  n195 = for {
    tunnel: w6 -> [w622] mode=indexing
    tunnel: w7 -> [w621] mode=indexing
    n196 = DataSocket Close(8:w621, 11:w622) -> ()  [unwired: 3 out]
  }
  n197 = for {
    tunnel: w32 -> [w626] mode=indexing
    tunnel: [w625] -> w29 mode=indexing
    tunnel: [w624] -> w28 mode=indexing
    n198 = DataSocket Open(10:T1."Read" ("mode"), 11:w626) -> (0:w624:errorcluster, 3:w625:refnum<k13>)  [unwired: 1 in, 1 out]
  }
  n199 = while {
    tunnel: w1 -> [w921]
    tunnel: w2 -> [w905]
    tunnel: [w877] -> w31
    tunnel: [w876] -> w30
    tunnel: w29 -> [w875]
    tunnel: w28 -> [w874]
    stop <- TRUE continue-if-true
    w658 = "\r"
    w647 = "\r"
    w636 = "\r"
    w687 = "\r"
    w699 = "\r"
    w711 = "\r"
    w723 = "\r"
    w735 = "\r"
    w747 = "\r"
    w759 = "\r"
    w771 = "\r"
    w783 = "\r"
    w795 = "\r"
    w807 = "\r"
    w819 = "\r"
    w831 = "\r"
    w843 = "\r"
    w855 = "\r"
    w867 = "\r"
    # "Reading PLC Actuation Values"
    n200 = for {
      tunnel: w875 -> [w928] mode=indexing
      tunnel: [w930] -> w876 mode=indexing
      tunnel: w874 -> [w927] mode=indexing
      tunnel: [w925] -> w904 mode=indexing
      tunnel: [w929] -> w877 mode=indexing
      n201 = DataSocket Read(8:w927, 9:500 ("ms timeout (10000)"), 10:0.0, 11:w928) -> (0:w929:errorcluster, 2:w925:dbl, 3:w930:refnum<k13>)  [unwired: 5 out]
    }
    n202 = Wait Until Next ms Multiple(millisecond multiple=u32 30000) -> ()  [unwired: 1 out]
    n203 = Build Array(w904) -> (w669:dbl[][])
    n204 = Index Array(array=w669, index (row)=0, index (col)=18 ("disabled index (col)")) -> (element=w631:dbl)
    n205 = Index Array(array=w669, index (row)=0, index (col)=15 ("disabled index (col)")) -> (element=w676:dbl)
    n206 = Index Array(array=w669, index (row)=0, index (col)=16 ("disabled index (col)")) -> (element=w633:dbl)
    n207 = Index Array(array=w669, index (row)=0, index (col)=17 ("disabled index (col)")) -> (element=w632:dbl)
    n208 = Index Array(array=w669, index (row)=0, index (col)=0 ("disabled index (col)")) -> (element=w856:dbl)
    n209 = Index Array(array=w669, index (row)=0, index (col)=1 ("disabled index (col)")) -> (element=w844:dbl)
    n210 = Index Array(array=w669, index (row)=0, index (col)=2 ("disabled index (col)")) -> (element=w832:dbl)
    n211 = Index Array(array=w669, index (row)=0, index (col)=3 ("disabled index (col)")) -> (element=w820:dbl)
    n212 = Index Array(array=w669, index (row)=0, index (col)=4 ("disabled index (col)")) -> (element=w808:dbl)
    n213 = Index Array(array=w669, index (row)=0, index (col)=5 ("disabled index (col)")) -> (element=w796:dbl)
    n214 = Index Array(array=w669, index (row)=0, index (col)=6 ("disabled index (col)")) -> (element=w784:dbl)
    n215 = Index Array(array=w669, index (row)=0, index (col)=7 ("disabled index (col)")) -> (element=w772:dbl)
    n216 = Index Array(array=w669, index (row)=0, index (col)=8 ("disabled index (col)")) -> (element=w760:dbl)
    n217 = Index Array(array=w669, index (row)=0, index (col)=9 ("disabled index (col)")) -> (element=w748:dbl)
    n218 = Index Array(array=w669, index (row)=0, index (col)=10 ("disabled index (col)")) -> (element=w736:dbl)
    n219 = Index Array(array=w669, index (row)=0, index (col)=11 ("disabled index (col)")) -> (element=w724:dbl)
    n220 = Index Array(array=w669, index (row)=0, index (col)=12 ("disabled index (col)")) -> (element=w712:dbl)
    n221 = Index Array(array=w669, index (row)=0, index (col)=13 ("disabled index (col)")) -> (element=w700:dbl)
    n222 = Index Array(array=w669, index (row)=0, index (col)=14 ("disabled index (col)")) -> (element=w688:dbl)
    n223 = Number To Fractional String(number=w832, precision (6)=i16 2) -> (F-format string=w836:string)  [unwired: 2 in]
    n224 = Number To Fractional String(number=w820, precision (6)=i16 2) -> (F-format string=w824:string)  [unwired: 2 in]
    n225 = Number To Fractional String(number=w808, precision (6)=i16 2) -> (F-format string=w812:string)  [unwired: 2 in]
    n226 = Number To Fractional String(number=w844, precision (6)=i16 2) -> (F-format string=w848:string)  [unwired: 2 in]
    n227 = Number To Fractional String(number=w796, precision (6)=i16 2) -> (F-format string=w800:string)  [unwired: 2 in]
    n228 = Number To Fractional String(number=w700, precision (6)=i16 2) -> (F-format string=w704:string)  [unwired: 2 in]
    n229 = Number To Fractional String(number=w772, precision (6)=i16 2) -> (F-format string=w776:string)  [unwired: 2 in]
    n230 = Number To Fractional String(number=w856, precision (6)=i16 2) -> (F-format string=w860:string)  [unwired: 2 in]
    n231 = Number To Fractional String(number=w748, precision (6)=i16 2) -> (F-format string=w752:string)  [unwired: 2 in]
    n232 = Number To Fractional String(number=w712, precision (6)=i16 2) -> (F-format string=w716:string)  [unwired: 2 in]
    n233 = Number To Fractional String(number=w760, precision (6)=i16 2) -> (F-format string=w764:string)  [unwired: 2 in]
    n234 = Number To Fractional String(number=w688, precision (6)=i16 2) -> (F-format string=w692:string)  [unwired: 2 in]
    n235 = Number To Fractional String(number=w724, precision (6)=i16 2) -> (F-format string=w728:string)  [unwired: 2 in]
    n236 = Number To Fractional String(number=w784, precision (6)=i16 2) -> (F-format string=w788:string)  [unwired: 2 in]
    n237 = Number To Fractional String(number=w676, precision (6)=i16 2) -> (F-format string=w680:string)  [unwired: 2 in]
    n238 = Number To Fractional String(number=w736, precision (6)=i16 2) -> (F-format string=w740:string)  [unwired: 2 in]
    n239 = Number To Fractional String(number=w633, precision (6)=i16 2) -> (F-format string=w643:string)  [unwired: 2 in]
    n240 = Number To Fractional String(number=w632, precision (6)=i16 2) -> (F-format string=w654:string)  [unwired: 2 in]
    n241 = Number To Fractional String(number=w631, precision (6)=i16 2) -> (F-format string=w665:string)  [unwired: 2 in]
    n242 = Format Date/Time String(time format string (%c)="%y%m%d%H%M%S") -> (date/time string=w835:string)  [unwired: 2 in]
    n243 = Format Date/Time String(time format string (%c)="%y%m%d%H%M%S") -> (date/time string=w823:string)  [unwired: 2 in]
    n244 = Format Date/Time String(time format string (%c)="%y%m%d%H%M%S") -> (date/time string=w811:string)  [unwired: 2 in]
    n245 = Format Date/Time String(time format string (%c)="%y%m%d%H%M%S") -> (date/time string=w847:string)  [unwired: 2 in]
    n246 = Format Date/Time String(time format string (%c)="%y%m%d%H%M%S") -> (date/time string=w799:string)  [unwired: 2 in]
    n247 = Format Date/Time String(time format string (%c)="%y%m%d%H%M%S") -> (date/time string=w703:string)  [unwired: 2 in]
    n248 = Format Date/Time String(time format string (%c)="%y%m%d%H%M%S") -> (date/time string=w775:string)  [unwired: 2 in]
    n249 = Format Date/Time String(time format string (%c)="%y%m%d%H%M%S") -> (date/time string=w859:string)  [unwired: 2 in]
    n250 = Format Date/Time String(time format string (%c)="%y%m%d%H%M%S") -> (date/time string=w751:string)  [unwired: 2 in]
    n251 = Format Date/Time String(time format string (%c)="%y%m%d%H%M%S") -> (date/time string=w715:string)  [unwired: 2 in]
    n252 = Format Date/Time String(time format string (%c)="%y%m%d%H%M%S") -> (date/time string=w763:string)  [unwired: 2 in]
    n253 = Format Date/Time String(time format string (%c)="%y%m%d%H%M%S") -> (date/time string=w691:string)  [unwired: 2 in]
    n254 = Format Date/Time String(time format string (%c)="%y%m%d%H%M%S") -> (date/time string=w727:string)  [unwired: 2 in]
    n255 = Format Date/Time String(time format string (%c)="%y%m%d%H%M%S") -> (date/time string=w787:string)  [unwired: 2 in]
    n256 = Format Date/Time String(time format string (%c)="%y%m%d%H%M%S") -> (date/time string=w679:string)  [unwired: 2 in]
    n257 = Format Date/Time String(time format string (%c)="%y%m%d%H%M%S") -> (date/time string=w739:string)  [unwired: 2 in]
    n258 = Format Date/Time String(time format string (%c)="%y%m%d%H%M%S") -> (date/time string=w644:string)  [unwired: 2 in]
    n259 = Format Date/Time String(time format string (%c)="%y%m%d%H%M%S") -> (date/time string=w655:string)  [unwired: 2 in]
    n260 = Format Date/Time String(time format string (%c)="%y%m%d%H%M%S") -> (date/time string=w666:string)  [unwired: 2 in]
    n261 = Concatenate Strings("2001" ("string"), w843, "A" ("string"), w843, "63" ("string"), w843, w836, w843, w835, w843, "LB201_A213", w843, "0.5524 0.3240 0.5" ("string")) -> (w833:string)
    "LB201_A213_SV201" <- w833
    n262 = Concatenate Strings("2001" ("string"), w831, "A" ("string"), w831, "65" ("string"), w831, w824, w831, w823, w831, "LB201_A213", w831, "0.5524 0.3240 0.5" ("string")) -> (w821:string)
    "LB201_A213_SV401" <- w821
    n263 = Concatenate Strings("2002" ("string"), w819, "A" ("string"), w819, "61" ("string"), w819, w812, w819, w811, w819, "LB201_A225", w819, "0.3145 0.3240 0.5" ("string")) -> (w809:string)
    "LB201_A225_ST901" <- w809
    n264 = Concatenate Strings("2001" ("string"), w855, "A" ("string"), w855, "62" ("string"), w855, w848, w855, w847, w855, "LB201_A213", w855, "0.5524 0.3240 0.5" ("string")) -> (w845:string)
    "LB201_A213_ST902" <- w845
    n265 = Concatenate Strings("2002" ("string"), w807, "A" ("string"), w807, "62" ("string"), w807, w800, w807, w799, w807, "LB201_A225", w807, "0.3145 0.3240 0.5" ("string")) -> (w797:string)
    "LB201_A225_ST902" <- w797
    n266 = Concatenate Strings("2004" ("string"), w711, "A" ("string"), w711, "62" ("string"), w711, w704, w711, w703, w711, "LB201_B230", w711, "0.2761 0.6773 0.5" ("string")) -> (w701:string)
    "LB201_B230_ST902" <- w701
    n267 = Concatenate Strings("2002" ("string"), w783, "A" ("string"), w783, "65" ("string"), w783, w776, w783, w775, w783, "LB201_A225", w783, "0.3145 0.3240 0.5" ("string")) -> (w773:string)
    "LB201_A225_SV401" <- w773
    n268 = Concatenate Strings("2001" ("string"), w867, "A" ("string"), w867, "61" ("string"), w867, w860, w867, w859, w867, "LB201_A213", w867, "0.5524 0.3240 0.5" ("string")) -> (w857:string)
    "LB201_A213_ST901" <- w857
    n269 = Concatenate Strings("2003" ("string"), w759, "A" ("string"), w759, "62" ("string"), w759, w752, w759, w751, w759, "LB201_A235", w759, "0.1735 0.3240 0.5" ("string")) -> (w749:string)
    "LB201_A235_ST902" <- w749
    n270 = Concatenate Strings("2004" ("string"), w723, "A" ("string"), w723, "61" ("string"), w723, w716, w723, w715, w723, "LB201_B230", w723, "0.2761 0.6773 0.5" ("string")) -> (w713:string)
    "LB201_B230_ST901" <- w713
    n271 = Concatenate Strings("2003" ("string"), w771, "A" ("string"), w771, "61" ("string"), w771, w764, w771, w763, w771, "LB201_A235", w771, "0.1735 0.3240 0.5" ("string")) -> (w761:string)
    "LB201_A235_ST901" <- w761
    n272 = Concatenate Strings("2004" ("string"), w699, "A" ("string"), w699, "63" ("string"), w699, w692, w699, w691, w699, "LB201_B230", w699, "0.2761 0.6773 0.5" ("string")) -> (w689:string)
    "LB201_B230_SV201" <- w689
    n273 = Concatenate Strings("2003" ("string"), w735, "A" ("string"), w735, "65" ("string"), w735, w728, w735, w727, w735, "LB201_A235", w735, "0.1735 0.3240 0.5" ("string")) -> (w725:string)
    "LB201_A235_SV401" <- w725
    n274 = Concatenate Strings("2002" ("string"), w795, "A" ("string"), w795, "63" ("string"), w795, w788, w795, w787, w795, "LB201_A225", w795, "0.3145 0.3240 0.5" ("string")) -> (w785:string)
    "LB201_A225_SV201" <- w785
    n275 = Concatenate Strings("2004" ("string"), w687, "A" ("string"), w687, "65" ("string"), w687, w680, w687, w679, w687, "LB201_B230", w687, "0.2761 0.6773 0.5" ("string")) -> (w677:string)
    "LB201_B230_SV401" <- w677
    n276 = Concatenate Strings("2003" ("string"), w747, "A" ("string"), w747, "63" ("string"), w747, w740, w747, w739, w747, "LB201_A235", w747, "0.1735 0.3240 0.5" ("string")) -> (w737:string)
    "LB201_A235_SV201" <- w737
    n277 = Concatenate Strings("2005" ("string"), w636, "A" ("string"), w636, "61" ("string"), w636, w643, w636, w644, w636, "LB201_B218", w636, "0.5844 0.6607 0.5" ("string")) -> (w646:string)
    "LB201_B218_ST901" <- w646
    n278 = Concatenate Strings("2005" ("string"), w647, "A" ("string"), w647, "62" ("string"), w647, w654, w647, w655, w647, "LB201_B218", w647, "0.5844 0.6607 0.5" ("string")) -> (w657:string)
    "LB201_B218_ST902" <- w657
    n279 = Concatenate Strings("2005" ("string"), w658, "A" ("string"), w658, "65" ("string"), w658, w665, w658, w666, w658, "LB201_B218", w658, "0.5844 0.6607 0.5" ("string")) -> (w668:string)
    "LB201_B218_SV401" <- w668
    n280 = Enqueue Element(queue=w905, element=w857, error in (no error)=w921) -> (error out=w920:errorcluster)  [unwired: 1 in, 2 out]
    n281 = Enqueue Element(queue=w905, element=w845, error in (no error)=w920) -> (error out=w919:errorcluster)  [unwired: 1 in, 2 out]
    n282 = Enqueue Element(queue=w905, element=w833, error in (no error)=w919) -> (error out=w918:errorcluster)  [unwired: 1 in, 2 out]
    n283 = Enqueue Element(queue=w905, element=w821, error in (no error)=w918) -> (error out=w917:errorcluster)  [unwired: 1 in, 2 out]
    n284 = Enqueue Element(queue=w905, element=w809, error in (no error)=w917) -> (error out=w916:errorcluster)  [unwired: 1 in, 2 out]
    n285 = Enqueue Element(queue=w905, element=w797, error in (no error)=w916) -> (error out=w915:errorcluster)  [unwired: 1 in, 2 out]
    n286 = Enqueue Element(queue=w905, element=w785, error in (no error)=w915) -> (error out=w914:errorcluster)  [unwired: 1 in, 2 out]
    n287 = Enqueue Element(queue=w905, element=w773, error in (no error)=w914) -> (error out=w913:errorcluster)  [unwired: 1 in, 2 out]
    n288 = Enqueue Element(queue=w905, element=w761, error in (no error)=w913) -> (error out=w912:errorcluster)  [unwired: 1 in, 2 out]
    n289 = Enqueue Element(queue=w905, element=w749, error in (no error)=w912) -> (error out=w911:errorcluster)  [unwired: 1 in, 2 out]
    n290 = Enqueue Element(queue=w905, element=w737, error in (no error)=w911) -> (error out=w910:errorcluster)  [unwired: 1 in, 2 out]
    n291 = Enqueue Element(queue=w905, element=w725, error in (no error)=w910) -> (error out=w909:errorcluster)  [unwired: 1 in, 2 out]
    n292 = Enqueue Element(queue=w905, element=w713, error in (no error)=w909) -> (error out=w908:errorcluster)  [unwired: 1 in, 2 out]
    n293 = Enqueue Element(queue=w905, element=w701, error in (no error)=w908) -> (error out=w907:errorcluster)  [unwired: 1 in, 2 out]
    n294 = Enqueue Element(queue=w905, element=w689, error in (no error)=w907) -> (error out=w906:errorcluster)  [unwired: 1 in, 2 out]
    n295 = Enqueue Element(queue=w905, element=w677, error in (no error)=w906) -> (queue out=w630:refnum<queue>, error out=w629:errorcluster)  [unwired: 1 in, 1 out]
    n296 = Enqueue Element(queue=w630, element=w646, error in (no error)=w629) -> (queue out=w628:refnum<queue>, error out=w634:errorcluster)  [unwired: 1 in, 1 out]
    n297 = Enqueue Element(queue=w628, element=w657, error in (no error)=w634) -> (queue out=w627:refnum<queue>, error out=w635:errorcluster)  [unwired: 1 in, 1 out]
    n298 = Enqueue Element(queue=w627, element=w668, error in (no error)=w635) -> ()  [unwired: 1 in, 3 out]
  }
  n299 = for {
    tunnel: w30 -> [w932] mode=indexing
    tunnel: w31 -> [w931] mode=indexing
    n300 = DataSocket Close(8:w931, 11:w932) -> ()  [unwired: 3 out]
  }
